vi "Diagnostic Measurement.vi"(8 "error in (no error)":errorcluster, 11 "CAP-USB-1 in":refnum<class "CAP-USB-1.lvclass">) -> (0 "error out":errorcluster, 3 "CAP-USB-1 out":refnum<class "CAP-USB-1.lvclass">)   [LabVIEW 2014, in "CAP-USB-1.lvlib" / "CAP-USB-1.lvclass"]
doc: "En base a los datos de promedio de los transductores el codigo analiza si el transductor esta cortado o sin conectar"
uses:
  CAP-USB-1.lvclass
  CAP-USB-1.lvclass/CAP-USB-1.ctl
  API/CAP-USB/CAP-USB.lvlib
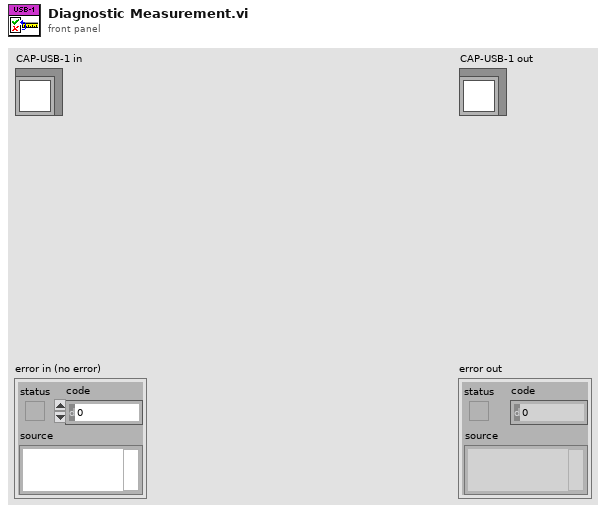
[diagram p1: front panel]
types:
  T1 = cluster{"Entradas":bool[], "Salidas":bool[], "Valor Encoder":u16, "Valor Transductores":u16[], "Orden Transd":u32[]}[]
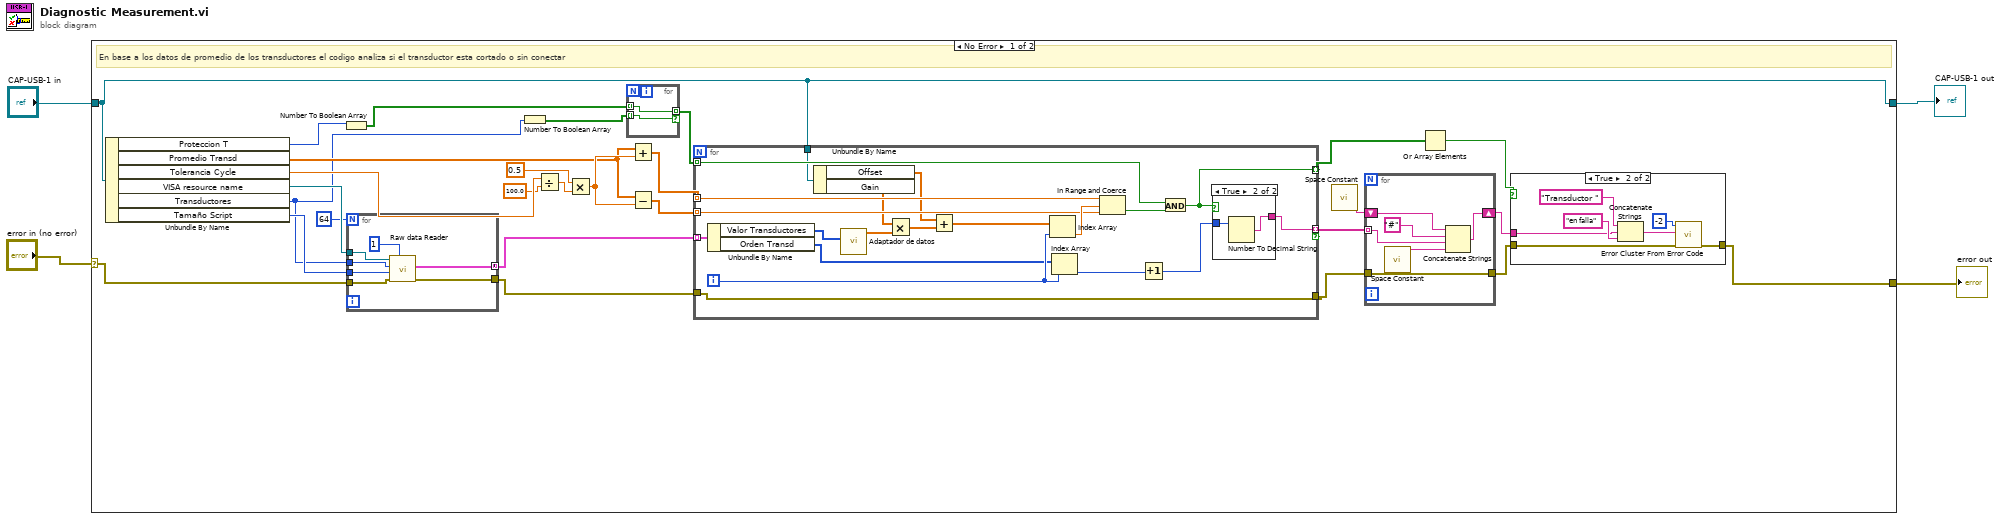
[diagram p0: block diagram]
diagram:
  n1 = case shown="No Error" "error in (no error)" {
    selector: "error in (no error)" -> [w24 w79]
    tunnel: [w18 w79] -> w3
    tunnel: [w5 w78] -> w1
    tunnel: "CAP-USB-1 in" -> [w5 w78]
    frame No Error {
      # "En base a los datos de promedio de los transductores el codigo analiza si el transductor esta cortado o sin conectar"
      n2 = Unbundle By Name(w5) -> ("Proteccion T"=w19:u64, "Promedio Transd"=w25:sgl[], "Tolerancia Cycle"=w32:sgl, "VISA resource name"=w21:refnum<visa-resource-name>, "Transductores"=w8:u64, "Tamaño Script"=w20:i32)
      n3 = Number To Boolean Array(number=w19) -> (Boolean array=w10:bool[])
      n4 = for {
        N: 64 -> [_]
        tunnel: [w37] -> w22 mode=concatenating
        tunnel: w21 -> [w36]
        tunnel: w20 -> [w35]
        tunnel: w8 -> [w34]
        tunnel: w24 -> [w39]
        tunnel: [w38] -> w23
        n5 = call "Raw data Reader.vi"("Num de tramas"=u32 1, "error in (no error)"=w39, "Tamaño Script"=w35, "TRANSDUCTORES"=w34, "VISA Refnum in"=w36) -> ("error out"=w38:errorcluster, "Raw data"=w37:T1)  [unwired: 2 in, 1 out]
      }
      n6 = Number To Boolean Array(number=w8) -> (Boolean array=w7:bool[])
      n7 = Divide(x=w32, y=sgl 100.0) -> (x/y=w30:sgl)
      n8 = Multiply(x=sgl 0.5, y=w30) -> (x*y=w26:sgl)
      n9 = for {
        tunnel: w10 -> [w41] mode=indexing
        tunnel: [w41] -> w9 mode=indexing if=w40
        tunnel: w7 -> [w40] mode=indexing
      }
      n10 = Add(x=w25, y=w26) -> (x+y=w28:sgl[])
      n11 = Subtract(x=w25, y=w26) -> (x-y=w27:sgl[])
      n12 = for {
        tunnel: w28 -> [w74] mode=indexing
        tunnel: w27 -> [w73] mode=indexing
        tunnel: w22 -> [w71] mode=indexing
        tunnel: w23 -> [w68]
        tunnel: w9 -> [w65] mode=indexing
        tunnel: [w68] -> w14
        tunnel: [w64] -> w17 mode=indexing
        tunnel: [w66] -> w12 mode=indexing if=w64
        tunnel: w5 -> [w61]
        i -> [w72]
        n13 = Unbundle By Name(w71) -> ("Valor Transductores"=w70:u16[], "Orden Transd"=w69:u32[])
        n14 = Unbundle By Name(w61) -> ("Offset"=w57:sgl[], "Gain"=w59:sgl[])
        n15 = call "Adaptador de datos.vi"("Transductores"=w70) -> ("Transductores"=w60:sgl[])  [unwired: 8 in, 2 out]
        n16 = Multiply(x=w59, y=w60) -> (x*y=w58:sgl[])
        n17 = Add(x=w57, y=w58) -> (x+y=w56:sgl[])
        n18 = Index Array(array=w56, index=w72) -> (element=w75:sgl)
        n19 = Index Array(array=w69, index=w72) -> (element=w63:u32)
        n20 = In Range and Coerce(upper limit=w74, x=w75, lower limit=w73) -> (In Range?=w67:bool)  [unwired: 1 out]
        n21 = Increment(x=w63) -> (x+1=w62:u32)
        n22 = And(x=w65, y=w67) -> (x .and. y?=w64:bool)
        n23 = case shown="True" w64 {
          tunnel: w62 -> [_ w77]
          tunnel: [_ w76] -> w66
          frame False {
          }
          frame True {
            n24 = Number To Decimal String(number=w77) -> (decimal integer string=w76:string)  [unwired: 1 in]
          }
        }
      }
      n25 = call <vilib>:"Space Constant.vi"() -> ("String"=w13:string)
      n26 = for {
        tunnel: [w47] -> w15
        tunnel: w14 -> [w47]
        shift-right: [w46] -> w11
        shift-left: w13 -> [w45]
        tunnel: w12 -> [w43] mode=indexing
        n27 = call <vilib>:"Space Constant.vi"() -> ("String"=w42:string)
        n28 = Concatenate Strings(w45, "#" ("string"), w43, w42) -> (w46:string)
      }
      n29 = Or Array Elements(Boolean array=w17) -> (logical OR=w16:bool)
      n30 = case shown="True" w16 {
        tunnel: w15 -> [w48 w51]
        tunnel: [w48 w50] -> w18
        tunnel: w11 -> [_ w49]
        frame False {
        }
        frame True {
          n31 = Concatenate Strings("Transductor ", w49, "en falla" ("string")) -> (w52:string)
          n32 = call <vilib>:"Error Cluster From Error Code.vi"("error in (no error)"=w51, "error message (\"\")"=w52, "error code (0)"=-2) -> ("error out"=w50:errorcluster)  [unwired: 6 in]
        }
      }
    }
    frame Error {
    }
  }
  "error out" <- w3
  "CAP-USB-1 out" <- w1
